vi "zeitgesteuerte schleife test.vi"() -> ()   [LabVIEW 2010]
uses:
  <vilib>/Platform/TimedLoop/XDataNode/nitl_modes.ctl
  <vilib>/Platform/TimedLoop/XDataNode/XDataNode.xnode
  <vilib>/Platform/TimedLoop/XDataNode/timing_clust.ctl
  <vilib>/Platform/TimedLoop/XDataNode/wakeup.ctl
  <vilib>/Platform/TimedLoop/XDataNode/loadnilvce.vi
  <vilib>/Platform/TimedLoop/XDataNode/XDNodeRunTimeDep.lvlib
panel:
  in  "Timeout":i32=-1
  in  "Frist":i64=-1
  in  "Priorität":i32=100
  out "Tatsächliches Ende [i-1]":i64
  out "Erwartetes Ende [i-1]":i64
  in  "Periode der Schleife":i64
  out "Verspätete Beendigung? [i-1]":bool
  in  "Count(mSec)":u32 caption="Anzahl (ms) warten"
  in  "Stopp":bool
  out "x/y":dbl
  in  "Modus":T1=enum."Discard missed periods, maintain original phase"
  out "x+y":i32
  in  "Fehler":errorcluster
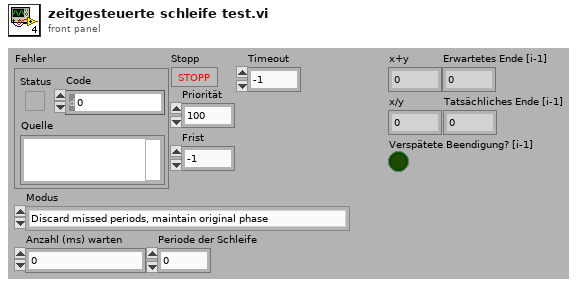
[diagram p1: front panel]
types:
  T1 = typedef "XDNodeRunTimeDep.lvlib/nitl_modes.ctl" = enum32{"No Change", "Process missed periods, maintain original phase", "Discard missed periods, maintain original phase", "Process missed periods, ignore original phase", "Discard missed periods, ignore original phase"}
  T2 = typedef "XDNodeRunTimeDep.lvlib/timing_clust.ctl" = cluster{"Expected End [f-1]":u64, "Actual End [f-1]":u64, "Finished Late? [f-1]":bool, "Expected End [i-1]":u64, "Actual End [i-1]":u64, "Finished Late? [i-1]":bool, "Expected Start [i]":u64, "Actual Start [i]":u64, "Expected Start [f]":u64, "Actual Start [f]":u64, "Source Name":string, "Structure Name":string, "Period":i64, "Deadline":i64, "Offset":i64, "Start":i64, "Priority":i32, "Timeout":i32, "Mode":T1, "Wakeup Reason":T3, "Error":errorcluster, "Source Type":string, "Secondary Source Type":string, "Global End Time":u64, "Global Start Time":u64, "Frame Duration":u64, "Iteration Duration":u64, "Assigned CPU":i32, "I/O Scan Engine Mode":u32}
  T3 = typedef "XDNodeRunTimeDep.lvlib/wakeup.ctl" = enum32{"Normal", "Aborted", "Asynchronous wakeup", "Timing source error", "Timed loop error", "Timeout"}
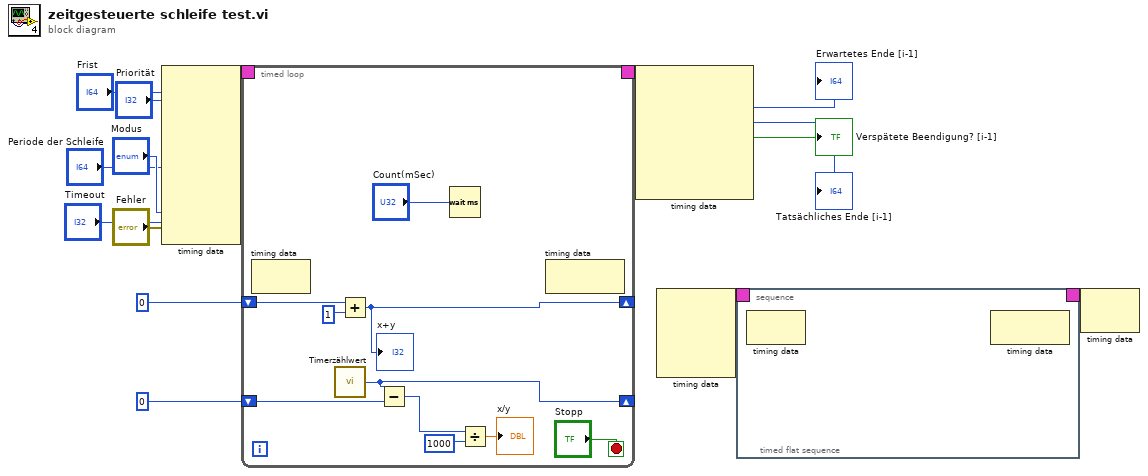
[diagram p0: block diagram]
diagram:
  n1 = node-c288("Frist", "Priorität", "Periode der Schleife", "Timeout", "Modus", "Fehler") -> (w15:T2)  [unwired: 4 in]
  n2 = timed-loop {
    timing: w15 -> [_]
    timing-out: [_] -> w14
    shift-right: [w23] -> _
    shift-left: 0 -> [w25]
    shift-right: [w18] -> _
    shift-left: u32 0 ("x") -> [w20]
    stop <- "Stopp" stop-if-true
    n3 = node-c288() -> ()  [unwired: 1 in, 1 out]
    n4 = call "Timerzählwert"() -> ("Tick Count(mSec)"=w18:u32)
    n5 = Add(x=w25, y=1) -> (x+y=w23:i32)
    "x+y" <- w23
    n6 = Subtract(x=w18, y=w20) -> (x-y=w19:u32)
    n7 = Wait (ms)(milliseconds to wait="Count(mSec)") -> ()  [unwired: 1 out]
    n8 = Divide(x=w19, y=u32 1000) -> (x/y=→"x/y":dbl)
    n9 = node-c288() -> ()  [unwired: 1 in, 1 out]
  }
  n10 = node-c288(w14) -> (→"Erwartetes Ende [i-1]":i64, →"Tatsächliches Ende [i-1]":i64, →"Verspätete Beendigung? [i-1]":bool)  [unwired: 4 out]
  n11 = node-c288() -> (w4:T2)  [unwired: 4 in]
  n12 = timed-sequence {
    timing: w4 -> [_]
    timing-out: [_] -> w3
    n13 = timed-flat-sequence {
      n14 = node-c288() -> ()  [unwired: 1 in, 1 out]
      n15 = node-c288() -> ()  [unwired: 1 in, 1 out]
    }
  }
  n16 = node-c288(w3) -> ()  [unwired: 1 out]
